vi "Continuity_DiodeTest.vi"(6 "Settling (s)":dbl format="%#_6p", 9 "PPMU_Parameters":T1, 10 "Pins":T2[](array[typedef]), 11 "Semiconductor Module Context":T3) -> (0 "error out":errorcluster)   [LabVIEW 2023, in "Continuity.lvlib"]
doc: "Continuity test by measuring the Voltage over protection diode"
uses:
  Continuity.lvlib
  <vilib>/NI_TestStand_SemiconductorModule/NI_TestStand_Semiconductor_Module.lvlibp/PinMap/General/SemiconductorModuleContext.ctl
  <vilib>/NI_TestStand_SemiconductorModule/NI_TestStand_Semiconductor_Module.lvlibp/PinMap/TagProvider/TSM_Pin.ctl
  ResourceHandling/TypeDefs/RH_PPMU_Parameters.ctl
  <instrlib>/niDigital/niDigital.llb/niDigital Output Function.ctl
  <instrlib>/niDigital/niDigital.llb/niDigital Measurement Type.ctl
  <vilib>/NI_TestStand_SemiconductorModule/NI_TestStand_Semiconductor_Module.lvlibp/PinMap/Digital Pattern/SingleSessionPinQueryContext/DigitalPatternSingleSessionPinQueryContext.lvclass
  C:/Program Files/National Instruments/LabVIEW 2023/vi.lib/NI_TestStand_SemiconductorModule/NI_TestStand_Semiconductor_Module.lvlibp/PinMap/PinQueryContext/PinQueryContext.lvclass
  <vilib>/NI_TestStand_SemiconductorModule/NI_TestStand_Semiconductor_Module.lvlibp/PinMap/Digital Pattern/PinsToNIDigitalPatternSession.vi
  <vilib>/NI_TestStand_SemiconductorModule/NI_TestStand_Semiconductor_Module.lvlibp/PinMap/General/Publish/PublishDataDouble1D.vi
  <vilib>/NI_TestStand_SemiconductorModule/NI_TestStand_Semiconductor_Module.lvlibp
  ResourceHandling/ResourceHandling.lvlib
  C:/Program Files/National Instruments/LabVIEW 2023/vi.lib/NI_TestStand_SemiconductorModule/NI_TestStand_Semiconductor_Module.lvlibp/PinMap/PinQueryContext/MultiplePinSingleSessionQueryContext/MultiplePinSingleSessionQueryContext.lvclass
  C:/Program Files/National Instruments/LabVIEW 2023/vi.lib/NI_TestStand_SemiconductorModule/NI_TestStand_Semiconductor_Module.lvlibp/PinMap/Digital Pattern/SingleSessionPinQueryContext/DigitalPatternSingleSessionPinQueryContext.lvclass
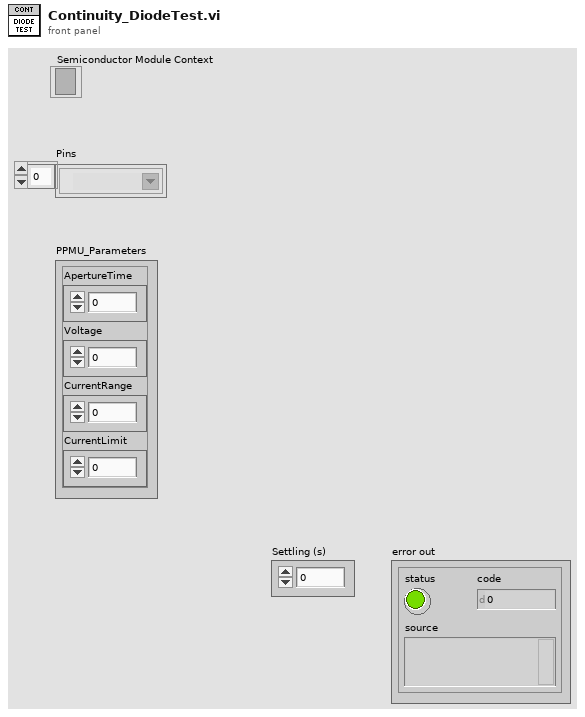
[diagram p1: front panel]
types:
  T1 = typedef "ResourceHandling.lvlib/RH_PPMU_Parameters.ctl" = cluster{"ApertureTime":dbl, "Voltage":dbl, "CurrentRange":dbl, "CurrentLimit":dbl}
  T2 = typedef "NI_TestStand_Semiconductor_Module.lvlibp/TSM_Pin.ctl" = tag
  T3 = typedef "NI_TestStand_Semiconductor_Module.lvlibp/SemiconductorModuleContext.ctl" = refnum<k7>
  T4 = typedef "niDigital Output Function.ctl" = i32
  T5 = typedef "niDigital Measurement Type.ctl" = i32
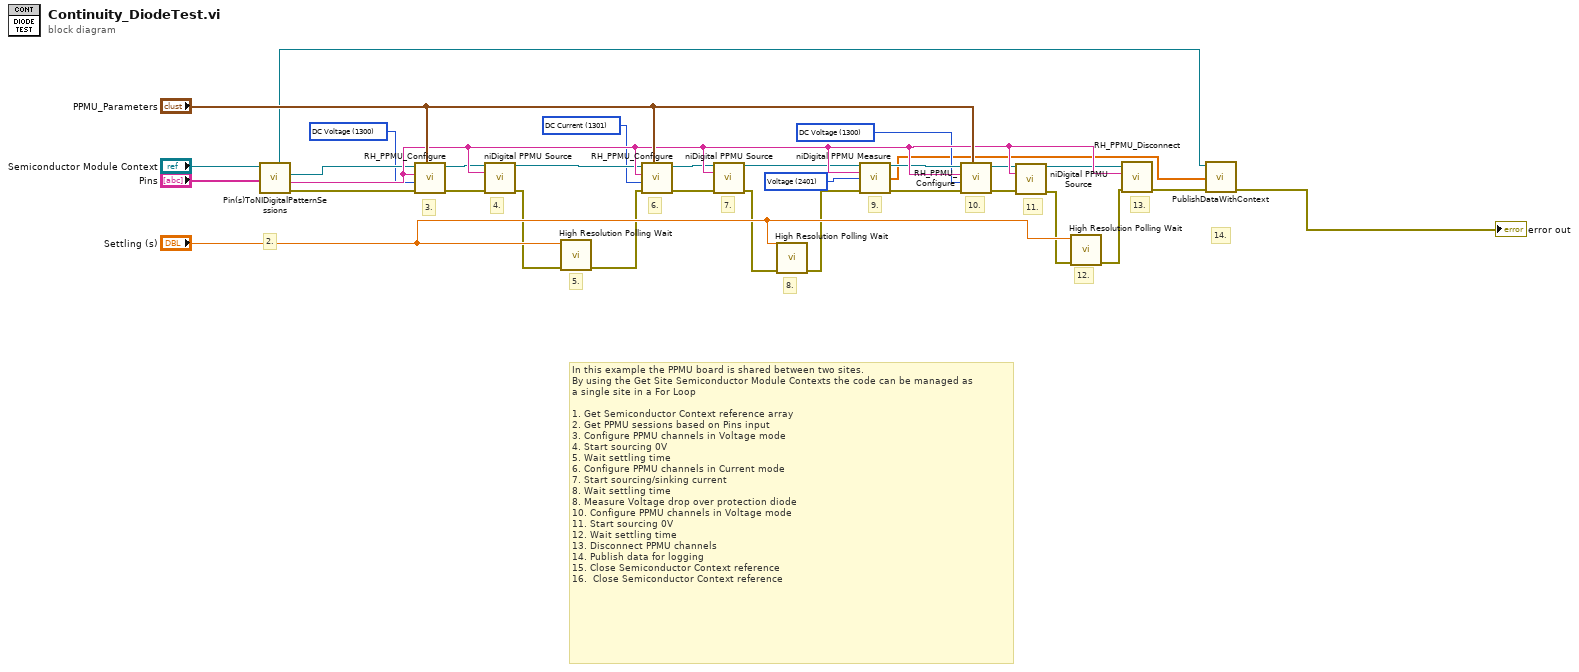
[diagram p0: block diagram]
diagram:
  w11 = T4 1300 items=["DC Voltage"=1300, "DC Current"=1301] ("output function")
  w14 = T5 2401 items=["Voltage"=2401, "Current"=2400] ("measurement type")
  w22 = T4 1301 items=["DC Voltage"=1300, "DC Current"=1301] ("output function")
  w26 = T4 1300 items=["DC Voltage"=1300, "DC Current"=1301] ("output function")
  # "14."
  # "13."
  # "12."
  # "11."
  # "10."
  # "9."
  # "8."
  # "7."
  # "6."
  # "5."
  # "4."
  # "3."
  # "2."
  # "In this example the PPMU board is shared between two sites.\nBy using the Get Site Semiconductor Module Contexts the code can be managed as\na single site in a For Loop\n\n1. Get Semiconductor Context reference array\n2. Get PPMU sessions based on Pins input\n3. Configure PPMU channels in Voltage mode\n4. Start sourcing 0V\n5. Wait settling time\n6. Configure PPMU channels in Current mode\n7. Start sourcing/sinking current\n8. Wait settling time\n8. Measure Voltage drop over protection diode\n10. Configure PPMU channels in Voltage mode\n11. Start sourcing 0V\n12. Wait settling time\n13. Disconnect PPMU channels\n14. Publish data for logging\n15. Close Semiconductor Context reference\n16.  Close Semiconductor Context reference"
  n1 = call-poly <vilib>:"Pin(s)ToNIDigitalPatternSessions.vi"("Pins"="Pins", "Semiconductor Module Context"="Semiconductor Module Context") -> ("error out"=w28:errorcluster, "Channel List"=w29:string, "Instrument Session"=w27:refnum<k15>, "Pin Query Context"=w2:refnum<class "DigitalPatternSingleSessionPinQueryContext.lvclass">)  [unwired: 4 in, 2 out]
  n2 = call "RH_PPMU_Configure.vi"("Digital_Parameters"="PPMU_Parameters", "error in"=w28, "output function"=w26, "channel list"=w29, "PPMU Session In"=w27) -> ("error out"=w24:errorcluster, "PPMU Session Out"=w25:refnum<k15>)  [unwired: 5 in]
  n3 = call <instrlib>:"niDigital PPMU Source.vi"("instrument handle"=w25, "channel list"=w29, "error in"=w24) -> ("instrument handle out"=w23:refnum<k15>, "error out"=w21:errorcluster)  [unwired: 11 in]
  n4 = call <vilib>:"High Resolution Polling Wait.vi"("error in (no error)"=w21, "seconds to wait"="Settling (s)") -> ("error out"=w20:errorcluster)  [unwired: 9 in]
  n5 = call "RH_PPMU_Configure.vi"("Digital_Parameters"="PPMU_Parameters", "error in"=w20, "output function"=w22, "channel list"=w29, "PPMU Session In"=w23) -> ("error out"=w18:errorcluster, "PPMU Session Out"=w19:refnum<k15>)  [unwired: 5 in]
  n6 = call <instrlib>:"niDigital PPMU Source.vi"("instrument handle"=w19, "channel list"=w29, "error in"=w18) -> ("instrument handle out"=w16:refnum<k15>, "error out"=w17:errorcluster)  [unwired: 11 in]
  n7 = call <vilib>:"High Resolution Polling Wait.vi"("error in (no error)"=w17, "seconds to wait"="Settling (s)") -> ("error out"=w15:errorcluster)  [unwired: 9 in]
  n8 = call <instrlib>:"niDigital PPMU Measure.vi"("instrument handle"=w16, "channel list"=w29, "measurement type"=w14, "error in"=w15) -> ("instrument handle out"=w12:refnum<k15>, "measurements"=w3:dbl[], "error out"=w13:errorcluster)  [unwired: 9 in]
  n9 = call "RH_PPMU_Configure.vi"("Digital_Parameters"="PPMU_Parameters", "error in"=w13, "output function"=w11, "channel list"=w29, "PPMU Session In"=w12) -> ("error out"=w9:errorcluster, "PPMU Session Out"=w10:refnum<k15>)  [unwired: 5 in]
  n10 = call <instrlib>:"niDigital PPMU Source.vi"("instrument handle"=w10, "channel list"=w29, "error in"=w9) -> ("instrument handle out"=w6:refnum<k15>, "error out"=w8:errorcluster)  [unwired: 11 in]
  n11 = call <vilib>:"High Resolution Polling Wait.vi"("error in (no error)"=w8, "seconds to wait"="Settling (s)") -> ("error out"=w7:errorcluster)  [unwired: 9 in]
  n12 = call "RH_PPMU_Disconnect.vi"("error in"=w7, "channel list"=w29, "PPMU Session In"=w6) -> ("error out"=w5:errorcluster)  [unwired: 7 in, 1 out]
  n13 = call-poly <vilib>:"PublishDataWithContext.vi"("error in (no error)"=w5, "Data In"=w3, "Pin Query Context"=w2) -> ("error out"=→"error out":errorcluster)  [unwired: 7 in, 1 out]
